vi "GSP_setmultiplecontrols.vi"(4 "error in (no error)":errorcluster, 6 "Control Infos":T1(array[cluster]), 7 "reference":refnum<vi>) -> (0 "error out":errorcluster, 3 "reference out":refnum<vi>)   [LabVIEW 2015]
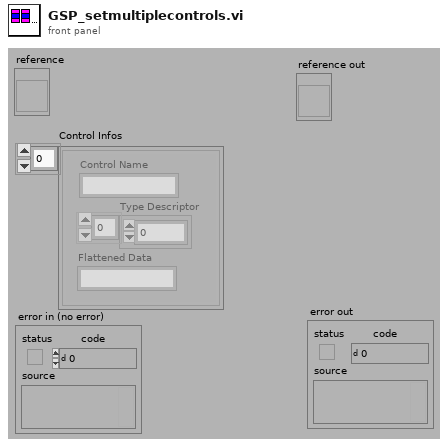
[diagram p1: front panel]
types:
  T1 = cluster{"Control Name":string, "Type Descriptor":i16[], "Flattened Data":string}[]
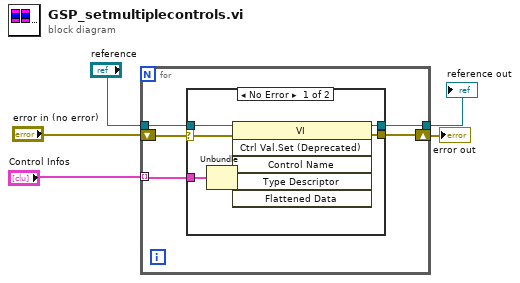
[diagram p0: block diagram]
diagram:
  n1 = for {
    tunnel: "Control Infos" -> [w6] mode=indexing
    shift-right: [w9] -> w3
    shift-left: "error in (no error)" -> [w10]
    tunnel: "reference" -> [w8]
    tunnel: [w7] -> w1
    n2 = case shown="No Error" w10 {
      selector: w10 -> [w18 w20]
      tunnel: [w17 w20] -> w9
      tunnel: w8 -> [w16 w19]
      tunnel: [w15 w19] -> w7
      tunnel: w6 -> [w14 _]
      frame No Error {
        n3 = Unbundle(w14) -> ("Control Name"=w13:string, "Type Descriptor"=w12:i16[], "Flattened Data"=w11:string)
        n4 = invoke class="VI" method="Ctrl Val.Set (Deprecated)"(reference=w16, error in=w18, "Control Name"=w13, "Type Descriptor"=w12, "Flattened Data"=w11) -> (reference out=w15:refnum<vi>, error out=w17:errorcluster)  [unwired: 1 in, 4 out]
      }
      frame Error {
      }
    }
  }
  "error out" <- w3
  "reference out" <- w1
